vi "Sandbox.vi"() -> ()   [LabVIEW 2019, in "NeedleValve.lvclass"]
uses:
  NeedleValve.lvclass
  TypeDef/Needle Valve Data.ctl
  modbus engine custom/MB_ENGINE_class/Engine State.ctl
  TypeDef/Needle Valve State.ctl
  modbus engine custom/MB_ENGINE_class/Engine Alarms.ctl
  modbus engine custom/MB_ENGINE_class/Settings.ctl
  modbus engine custom/MB_ENGINE_class/Limits Status.ctl
  TypeDef/Needle Valve Settings.ctl
  Database_Postgress_class/Database_Postgress.lvclass
  D:/GIT H4000/H4000/src/DatabaseInterface_class/DatabaseInterface.lvclass
  Database_Postgress_class/Connection Info.ctl
  Logger_class/Logger.lvclass
  ConfigJSON_class/ConfigJSON.lvclass
  D:/GIT H4000/H4000/src/ConfigInterface_class/ConfigInterface.lvclass
  MessageAMC_class/MessageAMC.lvclass
  D:/GIT H4000/H4000/src/MessageInterface_class/MessageInterface.lvclass
  ConfigJSON_class/ConfigJSON.lvclass/ConfigJSON.ctl
  SV_Puplisher_class/SV_Publisher.lvclass
  DatabaseInterface_class/DatabaseInterface.lvclass
  MessageInterface_class/MessageInterface.lvclass
  <vilib>/NI/AMC/AMC.lvlib
  modbus engine custom/MB_ENGINE_class/MB_ENGINE.lvclass
panel:
  in  "Needle Valve Settings":T1={"average size"=0, "open force"=12, "close force"=12, "open settings"={"ACC Steps Per Sec^2"=0, "DEC Steps Per Sec^2"=0, "Min Velosity Step Per Sec"=0, "Max Velosity Step Per Sec"=0, "MicroStep"=0}, "close settings"={"ACC Steps Per Sec^2"=0, "DEC Steps Per Sec^2"=0, "Min Velosity Step Per Sec"=0, "Max Velosity Step Per Sec"=0, "MicroStep"=0}}
  out "NVM_1_DATA":T3={"Engine State"=8, "StateValveModbus"=enum."IDLE", "Alarms"={"OL"=FALSE, "TF"=FALSE, "STL"=FALSE, "OCP"=FALSE, "CPUV"=FALSE, "UVLO"=FALSE, "SPI_ERROR"=FALSE, "Fault"=FALSE, "OL 2"=FALSE, "TF 2"=FALSE, "STL 2"=FALSE, "OCP 2"=FALSE, "CPUV 2"=FALSE, "UVLO 2"=FALSE, "reserved"=TRUE, "InitDone"=TRUE}, "RAW Possition"=124110, "Angele"=0.0, "Step"=0, "Encoder"=0, "Kinematic"={"ACC Steps Per Sec^2"=100, "DEC Steps Per Sec^2"=100, "Min Velosity Step Per Sec"=100, "Max Velosity Step Per Sec"=200, "MicroStep"=16}, "Limits"={"Fault 2 Switch"=FALSE, "Fault 1 Switch"=FALSE, "Center(Home)"=FALSE, "Lower Limit"=FALSE, "Upper Limit"=FALSE}} {"Engine State" items=["ACCELERATING", "DECELERATINGTOSTOP", "DECELERATING", "STEADY", "INDEX_ACCEL", "NDEX_RUN", "INDEX_DECEL", "INDEX_DWELL", "INACTIVE", "STANDBY", "STANDBYTOINACTIVE"]}
  in  "SET_SETTINGS":bool
  in  "clear":bool
  in  "stop":bool
  in  "close":bool
  in  "open":bool
  out "UDP port used":u16
  out "error out 2":errorcluster
  out "error out":errorcluster
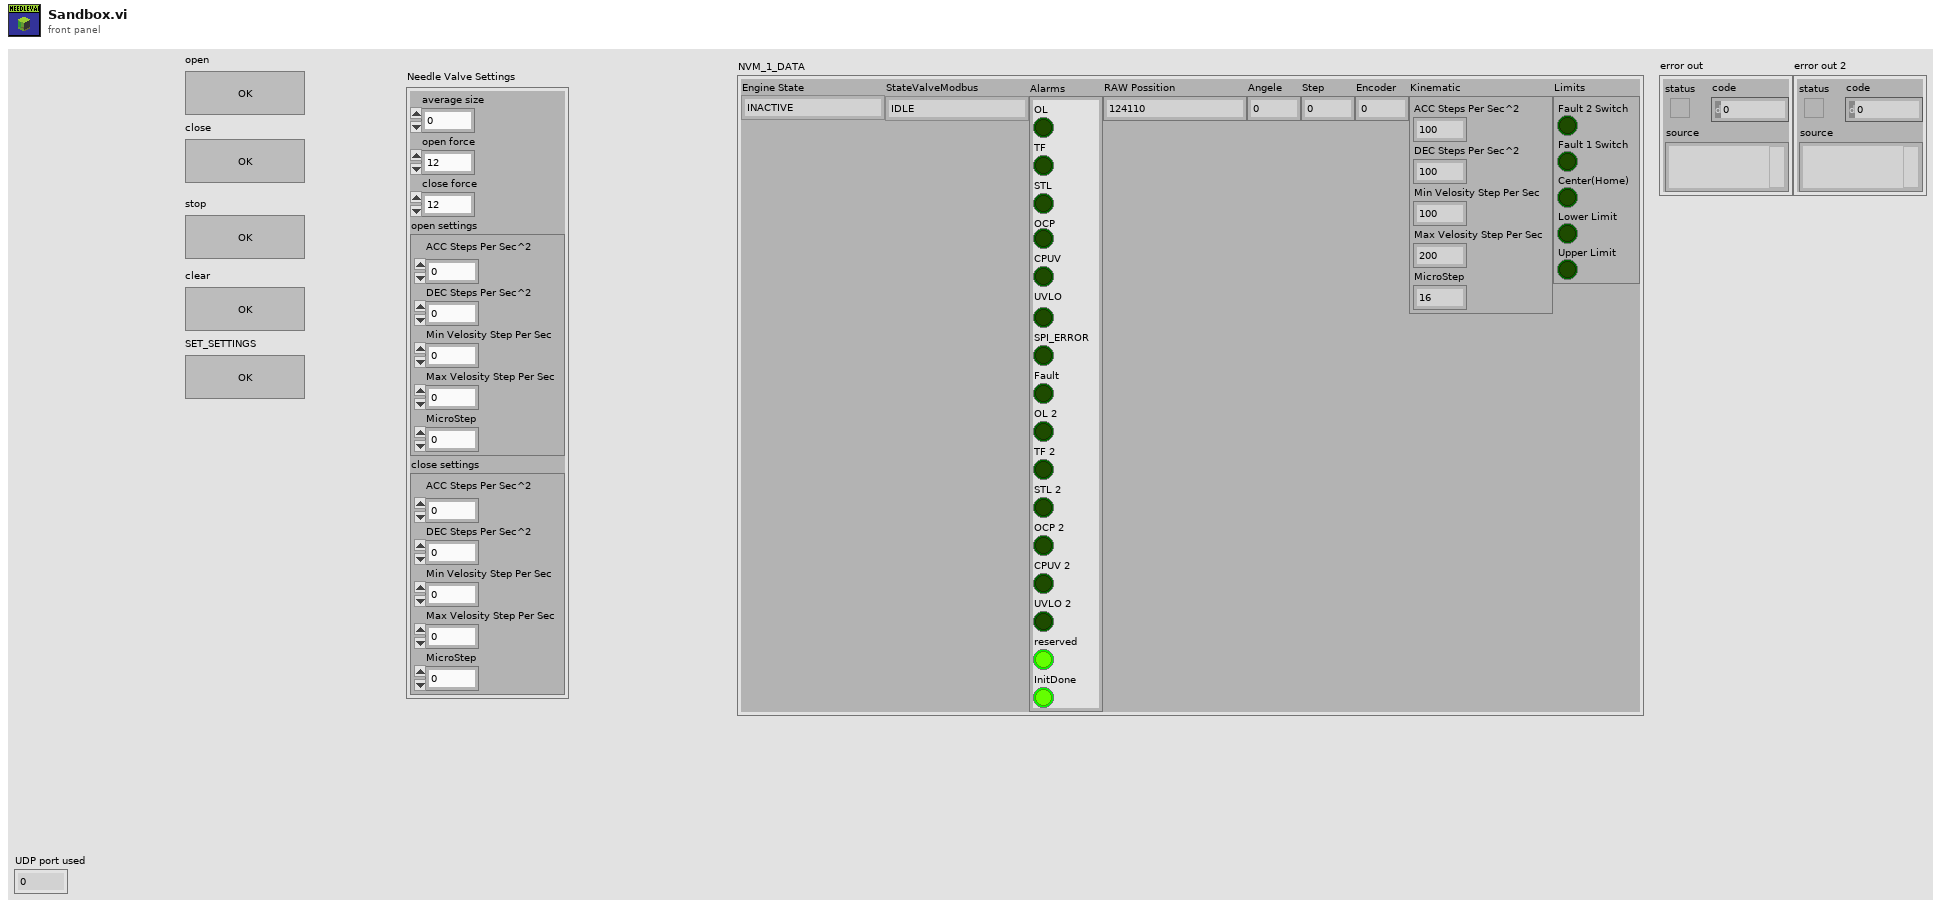
[diagram p1: front panel]
types:
  T1 = typedef "Needle Valve Settings.ctl" = cluster{"average size":i32, "open force":u16, "close force":u16, "open settings":T2, "close settings":T2}
  T2 = typedef "MB_ENGINE.lvclass/Settings.ctl" = cluster{"ACC Steps Per Sec^2":u16, "DEC Steps Per Sec^2":u16, "Min Velosity Step Per Sec":u16, "Max Velosity Step Per Sec":u16, "MicroStep":u16}
  T3 = typedef "Needle Valve Data.ctl" = cluster{"Engine State":T4, "StateValveModbus":T5, "Alarms":T6, "RAW Possition":i32, "Angele":dbl, "Step":i32, "Encoder":i32, "Kinematic":T2, "Limits":T7}
  T4 = typedef "MB_ENGINE.lvclass/Engine State.ctl" = u16
  T5 = typedef "Needle Valve State.ctl" = enum16{"IDLE", "OPENING", "CLOSING", "STOP"}
  T6 = typedef "MB_ENGINE.lvclass/Engine Alarms.ctl" = cluster{"OL":bool, "TF":bool, "STL":bool, "OCP":bool, "CPUV":bool, "UVLO":bool, "SPI_ERROR":bool, "Fault":bool, "OL 2":bool, "TF 2":bool, "STL 2":bool, "OCP 2":bool, "CPUV 2":bool, "UVLO 2":bool, "reserved":bool, "InitDone":bool}
  T7 = typedef "MB_ENGINE.lvclass/Limits Status.ctl" = cluster{"Fault 2 Switch":bool, "Fault 1 Switch":bool, "Center(Home)":bool, "Lower Limit":bool, "Upper Limit":bool}
  T8 = typedef "DatabaseInterface.lvclass/Connection Info.ctl" = cluster{"IP_Address":string, "Port":u16, "Timeout":i32, "User":string, "Password":string, "Database":string}
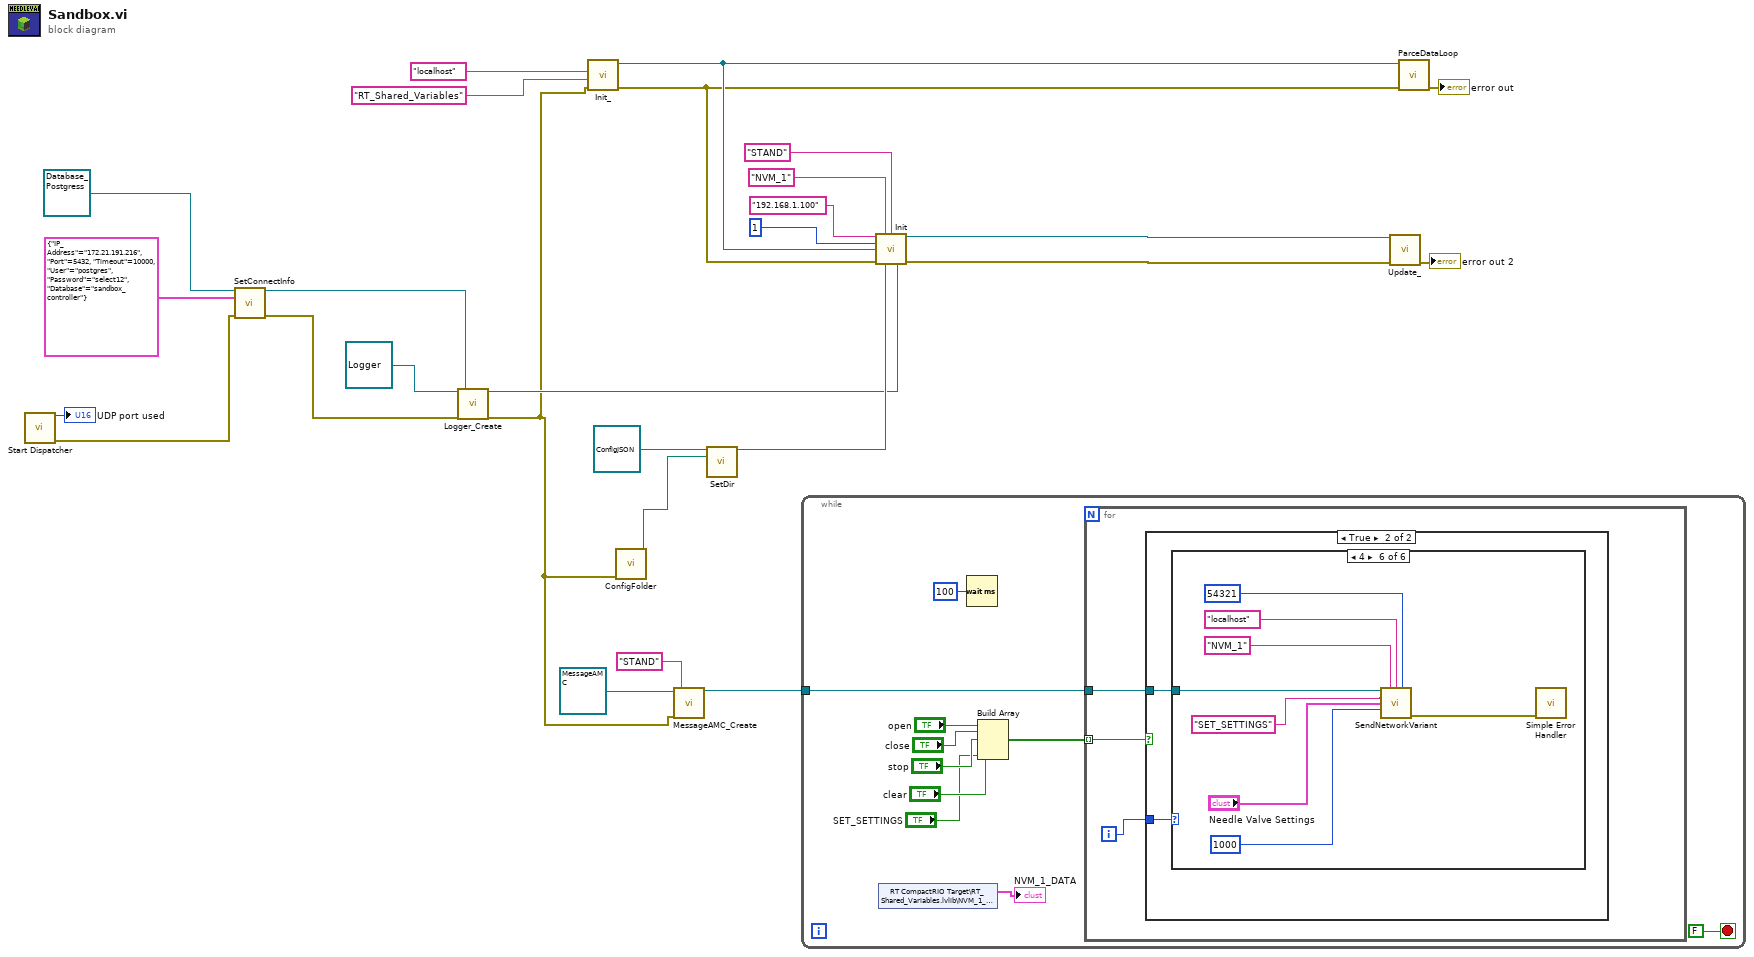
[diagram p0: block diagram]
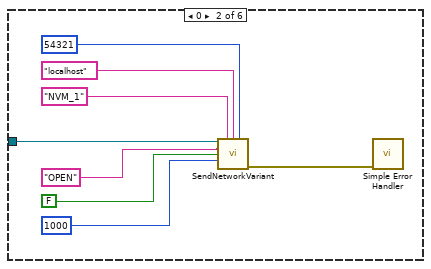
[diagram p4: hidden frame]
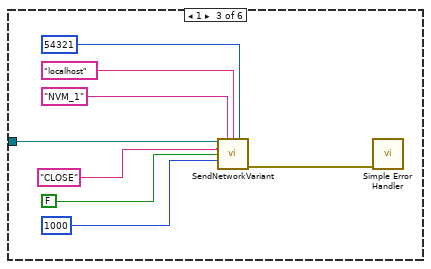
[diagram p5: hidden frame]
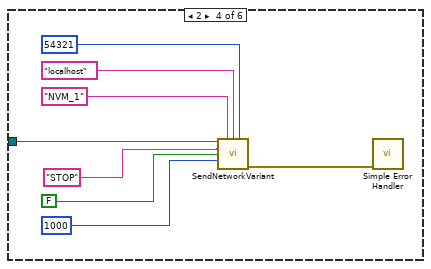
[diagram p6: hidden frame]
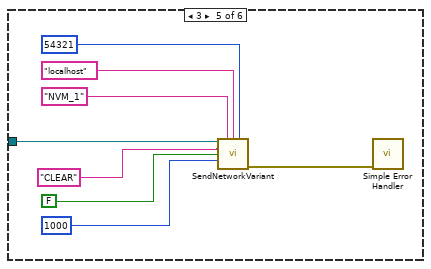
[diagram p7: hidden frame]
diagram:
  n1 = call <vilib>:"Start Dispatcher.vi"() -> ("UDP port used"=→"UDP port used":u16, "error out"=w5:errorcluster)  [unwired: 13 in, 1 out]
  n2 = call-dynamic "SetConnectInfo.vi"("reference in"=refnum<class "Database_Postgress.lvclass"> refnum, "Connection Info"=T8 {"IP_Address"="172.21.191.216", "Port"=5432, "Timeout"=10000, "User"="postgres", "Password"="select12", "Database"="sandbox_controller"}, "error in (no error)"=w5) -> ("reference out"=w15:refnum<class "Database_Postgress.lvclass">, "error out"=w14:errorcluster)  [unwired: 11 in]
  n3 = call "Logger_Create.vi"("reference in"=refnum<class "Logger.lvclass"> refnum, "error in (no error)"=w14, "DatabaseInterface"=w15) -> ("reference out"=w10:refnum<class "Logger.lvclass">, "error out"=w1:errorcluster)  [unwired: 15 in]
  n4 = call "Init_.vi"("error in (no error)"=w1, "lib"="RT_Shared_Variables", "host"="localhost") -> ("error out"=w19:errorcluster, "SV_Publisher out"=w20:refnum<class "SV_Publisher.lvclass">)  [unwired: 7 in]
  n5 = call "ConfigFolder.vi"("error in (no error)"=w1) -> ("dup path"=w12:path)  [unwired: 13 in, 1 out]
  n6 = call "MessageAMC_Create.vi"("reference in"=refnum<class "MessageAMC.lvclass"> refnum ("MessageAMC"), "error in (no error)"=w1, "message queue name"="STAND") -> ("amc"=w3:refnum<class "MessageAMC.lvclass">)  [unwired: 15 in, 1 out]
  n7 = call "SetDir.vi"("reference in"=refnum<class "ConfigJSON.lvclass"> refnum ("ConfigJSON"), "Config Dir"=w12) -> ("JSON"=w11:refnum<class "ConfigJSON.lvclass">)  [unwired: 13 in]
  n8 = while {
    tunnel: w3 -> [w37]
    stop <- FALSE stop-if-true
    n9 = shared-variable "RT CompactRIO Target\\RT_Shared_Variables.lvlib\\NVM_1_DATA"() -> (→"NVM_1_DATA":T3)  [unwired: 1 in, 1 out]
    n10 = Wait (ms)(milliseconds to wait=u32 100) -> ()  [unwired: 1 out]
    n11 = Build Array("open", "close", "stop", "clear", "SET_SETTINGS") -> (w31:bool[])
    n12 = for {
      tunnel: w37 -> [w40]
      tunnel: w31 -> [w39] mode=indexing
      i -> [w38]
      n13 = case shown="True" w39 {
        tunnel: w40 -> [_ w42]
        tunnel: w38 -> [_ w41]
        frame False {
        }
        frame True {
          n14 = case shown="4" w41 {
            tunnel: w42 -> [_ w44 w52 w60 w68 w77]
            frame Default {
            }
            frame 0 {
              n15 = call "SendNetworkVariant.vi"("reference in"=w44, "receiver process"="NVM_1", "receiver host"="localhost", "receiver port (0)"=u16 54321, "name"="OPEN", "data"=FALSE, "timeout (25000 ms)"=1000) -> ("error out"=w48:errorcluster)  [unwired: 6 in, 2 out]
              n16 = call <vilib>:"Simple Error Handler.vi"("error in (no error)"=w48) -> ()  [unwired: 4 in, 5 out]
            }
            frame 1 {
              n17 = call "SendNetworkVariant.vi"("reference in"=w52, "receiver process"="NVM_1", "receiver host"="localhost", "receiver port (0)"=u16 54321, "name"="CLOSE", "data"=FALSE, "timeout (25000 ms)"=1000) -> ("error out"=w56:errorcluster)  [unwired: 6 in, 2 out]
              n18 = call <vilib>:"Simple Error Handler.vi"("error in (no error)"=w56) -> ()  [unwired: 4 in, 5 out]
            }
            frame 2 {
              n19 = call "SendNetworkVariant.vi"("reference in"=w60, "receiver process"="NVM_1", "receiver host"="localhost", "receiver port (0)"=u16 54321, "name"="STOP", "data"=FALSE, "timeout (25000 ms)"=1000) -> ("error out"=w64:errorcluster)  [unwired: 6 in, 2 out]
              n20 = call <vilib>:"Simple Error Handler.vi"("error in (no error)"=w64) -> ()  [unwired: 4 in, 5 out]
            }
            frame 3 {
              n21 = call "SendNetworkVariant.vi"("reference in"=w68, "receiver process"="NVM_1", "receiver host"="localhost", "receiver port (0)"=u16 54321, "name"="CLEAR", "data"=FALSE, "timeout (25000 ms)"=1000) -> ("error out"=w72:errorcluster)  [unwired: 6 in, 2 out]
              n22 = call <vilib>:"Simple Error Handler.vi"("error in (no error)"=w72) -> ()  [unwired: 4 in, 5 out]
            }
            frame 4 {
              n23 = call "SendNetworkVariant.vi"("reference in"=w77, "receiver process"="NVM_1", "receiver host"="localhost", "receiver port (0)"=u16 54321, "name"="SET_SETTINGS", "data"="Needle Valve Settings", "timeout (25000 ms)"=1000) -> ("error out"=w80:errorcluster)  [unwired: 6 in, 2 out]
              n24 = call <vilib>:"Simple Error Handler.vi"("error in (no error)"=w80) -> ()  [unwired: 4 in, 5 out]
            }
          }
        }
      }
    }
  }
  n25 = call "Init.vi"("address"="192.168.1.100", "Name"="NVM_1", "ParentName"="STAND", "addres"=u16 1, "SV_Publisher"=w20, "error in (no error)"=w19, "ConfigInterface"=w11, "Logger"=w10) -> ("NeedleValve out"=w9:refnum<class "NeedleValve.lvclass">, "error out"=w8:errorcluster)  [unwired: 6 in]
  n26 = call "Update_.vi"("Pump_1AI_1DO_2DI in"=w9, "error in (no error)"=w8) -> ("error out"=→"error out 2":errorcluster)  [unwired: 12 in, 1 out]
  n27 = call "ParceDataLoop.vi"("error in (no error)"=w19, "SV_Publisher in"=w20) -> ("error out"=→"error out":errorcluster)  [unwired: 9 in]
